vi "REQUEST_DATA_STREAM.vi"(10 "Payload":T1={"req_message_rate"=10, "target_system"=0, "target_component"=0, "req_stream_id"=enum."ALL", "start_stop"=FALSE}) -> (3 "MAVLink MSG":u8[](array[numeric]))   [LabVIEW 2014]
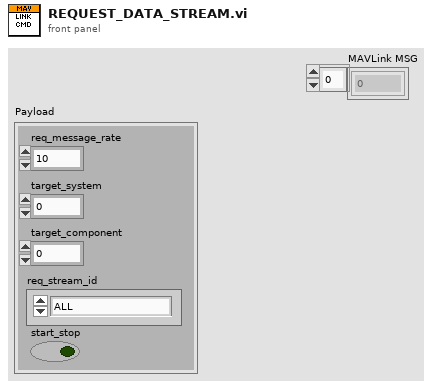
[diagram p1: front panel]
types:
  T1 = cluster{"req_message_rate":u16, "target_system":u8, "target_component":u8, "req_stream_id":enum16{"ALL", "RAW_SENSORS", "EXTENDED_STATUS", "RC_CHANNELS", "RAW_CONTROLLER", "POSITION", "EXTRA1", "EXTRA2", "EXTRA3"}, "start_stop":bool}
  T2 = enum16{"ALL", "RAW_SENSORS", "EXTENDED_STATUS", "RC_CHANNELS", "RAW_CONTROLLER", "POSITION", "EXTRA1", "EXTRA2", "EXTRA3"}
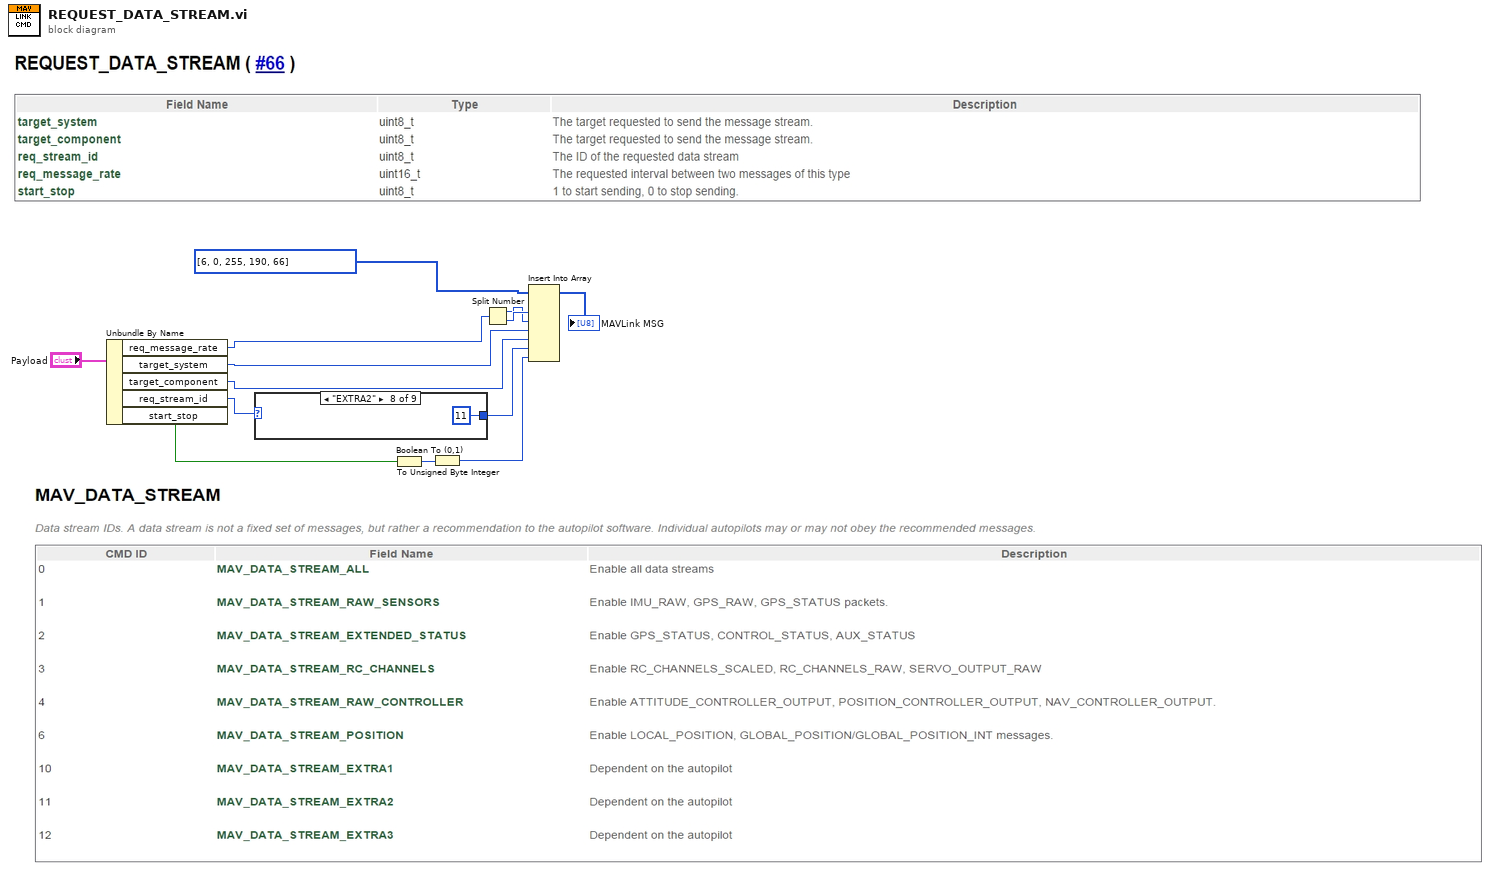
[diagram p0: block diagram]
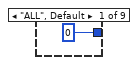
[diagram p2: hidden frame]
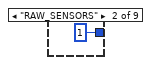
[diagram p3: hidden frame]
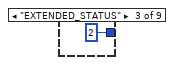
[diagram p4: hidden frame]
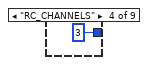
[diagram p5: hidden frame]
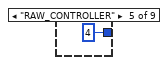
[diagram p6: hidden frame]
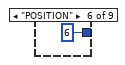
[diagram p7: hidden frame]
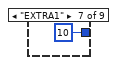
[diagram p8: hidden frame]
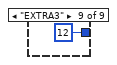
[diagram p9: hidden frame]
diagram:
  n1 = Unbundle By Name("Payload") -> ("req_message_rate"=w10:u16, "target_system"=w9:u8, "target_component"=w8:u8, "req_stream_id"=w4:T2, "start_stop"=w7:bool)
  n2 = case shown="\"EXTRA2\"" w4 {
    tunnel: [u8 0 ("unsigned 8bit integer") u8 1 ("unsigned 8bit integer") u8 2 ("unsigned 8bit integer") u8 3 ("unsigned 8bit integer") u8 4 ("unsigned 8bit integer") u8 6 ("unsigned 8bit integer") u8 10 ("unsigned 8bit integer") u8 11 ("unsigned 8bit integer") u8 12 ("unsigned 8bit integer")] -> w3
    frame "ALL", Default {
    }
    frame "RAW_SENSORS" {
    }
    frame "EXTENDED_STATUS" {
    }
    frame "RC_CHANNELS" {
    }
    frame "RAW_CONTROLLER" {
    }
    frame "POSITION" {
    }
    frame "EXTRA1" {
    }
    frame "EXTRA2" {
    }
    frame "EXTRA3" {
    }
  }
  n3 = Boolean To (0,1)(Boolean=w7) -> (0, 1=w13:i16)
  n4 = To Unsigned Byte Integer(number=w13) -> (unsigned 8bit integer=w12:u8)
  n5 = Split Number(x=w10) -> (hi(x)=w1:u8, lo(x)=w2:u8)
  n6 = Insert Into Array(array=u8[] [6, 0, 255, 190, 66], new element #1=w2, new element #2=w1, new element #3=w9, new element #4=w8, new element #5=w3, new element #6=w12) -> (→"MAVLink MSG":u8[])  [unwired: 1 in]
